vi "CoboltLaser_ModeGet.vi"(0 "ComPort":refnum<visa-resource-name>, 7 "CheckResponse":bool=TRUE, 11 "ErrorIn":errorcluster) -> (4 "ComPortOut":refnum<visa-resource-name>, 6 "Mode":T1 caption="Laser Mode", 8 "Response":string, 10 "Units(mA:1)":bool, 15 "ErrorOut":errorcluster)   [LabVIEW 2019]
doc: "Use this template to build a VI to use as a subVI."
uses:
  Programmes Labview/LabScanV1A/DevicesClass/InstrumentsClass/CoboltMLD/CoboltModes.ctl
panel:
  out "ResponseOK":bool
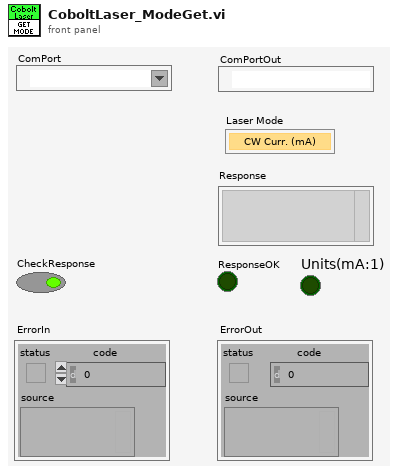
[diagram p1: front panel]
types:
  T1 = typedef "CoboltModes.ctl" = enum16{"CW Curr. (mA)", "CW Pow. (mW)", "Curr. Mod. (mA)", "Pow. Mod. (mW)"}
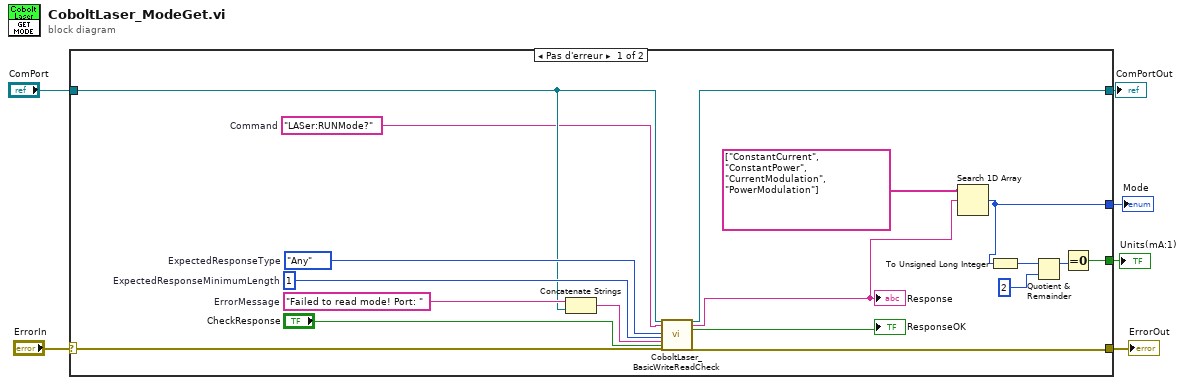
[diagram p0: block diagram]
diagram:
  n1 = case shown="Pas d'erreur" "ErrorIn" {
    selector: "ErrorIn" -> [w24 w26]
    tunnel: [w23 w26] -> w5
    tunnel: "ComPort" -> [w16 w25]
    tunnel: [w15 w25] -> w3
    tunnel: [w9 _] -> w2
    tunnel: [w7 _] -> w1
    frame No Error {
      w21 = 1  # ExpectedResponseMinimumLength
      w22 = enum16{"Any", "Digits Only", "Non-Digits Only"}."Any"  # ExpectedResponseType
      w18 = "Failed to read mode! Port: "  # ErrorMessage
      w14 = "LASer:RUNMode?"  # Command
      n2 = Concatenate Strings(w18, w16) -> (w17:string)
      n3 = call <userlib>:"CoboltLaser_BasicWriteReadCheck.vi"("ComPort"=w16, "Command"=w14, "ExpectedResponseType"=w22, "ExpectedResponseMinimumLength"=w21, "ErrorMessage"=w17, "GenerateError"="CheckResponse", "error in (no error)"=w24) -> ("ComPortOut"=w15:refnum<visa-resource-name>, "Response"=w12:string, "ResponseOK"=→"ResponseOK":bool, "error out"=w23:errorcluster)  [unwired: 17 in]
      "Response" <- w12
      n4 = Search 1D Array(1D array=string[] ["ConstantCurrent", "ConstantPower", "CurrentModulation", "PowerModulation"], element=w12) -> (index of element=w9:i32)  [unwired: 1 in]
      n5 = To Unsigned Long Integer(number=w9) -> (unsigned 32bit integer=w11:u32)
      n6 = Quotient & Remainder(x=w11, y=u32 2) -> (x-y*floor(x/y)=w8:u32)  [unwired: 1 out]
      n7 = Equal To 0?(x=w8) -> (x = 0?=w7:bool)
    }
    frame Error {
    }
  }
  "ErrorOut" <- w5
  "ComPortOut" <- w3
  "Mode" <- w2
  "Units(mA:1)" <- w1
